vi "Child Turn Compare.vi"(10 "Image Value from Second Move":dbl, 11 "Image value from First Move":dbl) -> (2 "Next Move":T1(ring))   [LabVIEW 2018]
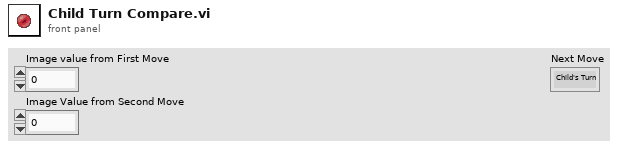
[diagram p1: front panel]
types:
  T1 = enum16{"Child's Turn", "Robot's Turn", "Waiting State", "Game Over"}
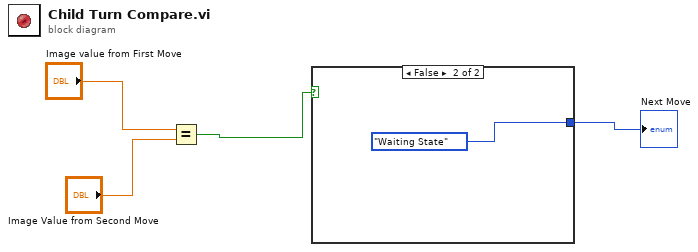
[diagram p0: block diagram]
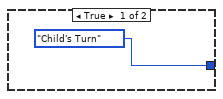
[diagram p2: hidden frame]
diagram:
  n1 = Equal?(x="Image value from First Move", y="Image Value from Second Move") -> (x = y?=w4:bool)
  n2 = case shown="False" w4 {
    tunnel: [T1."Child's Turn" T1."Waiting State"] -> w1
    frame True {
    }
    frame False {
    }
  }
  "Next Move" <- w1
